vi "tester.vi"() -> ()   [LabVIEW 2020]
uses:
  <vilib>/Utility/miscctls.llb/LVSelectionTypeDef.ctl
panel:
  out "Missmatches 3":T1[](array[typedef])
  out "Common":string="asssd"
  out "Missmatches 2":T1[](array[typedef])
  in  "Reference":string="asd"
  in  "Target":string="asssd"
  in  "String":string
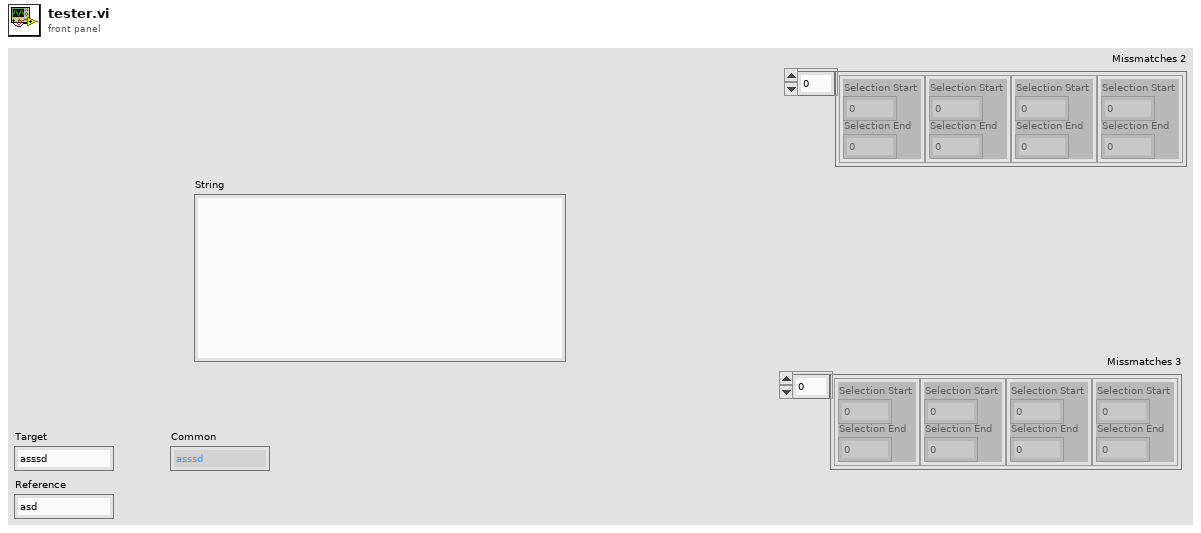
[diagram p1: front panel]
types:
  T1 = typedef "LVSelectionTypeDef.ctl" = cluster{"Selection Start":u32, "Selection End":u32}
  T2 = cluster{"Text.Selection":T1, "Text.Text Colors:Text Color":u32}[]
  T3 = cluster{"Selection Start":u32, "Selection End":u32}[]
  T4 = cluster{"Text.Selection":cluster{"Selection Start":u32, "Selection End":u32}, "Text.Text Colors:Text Color":u32}
  T5 = cluster{"Selection Start":u32, "Selection End":u32}
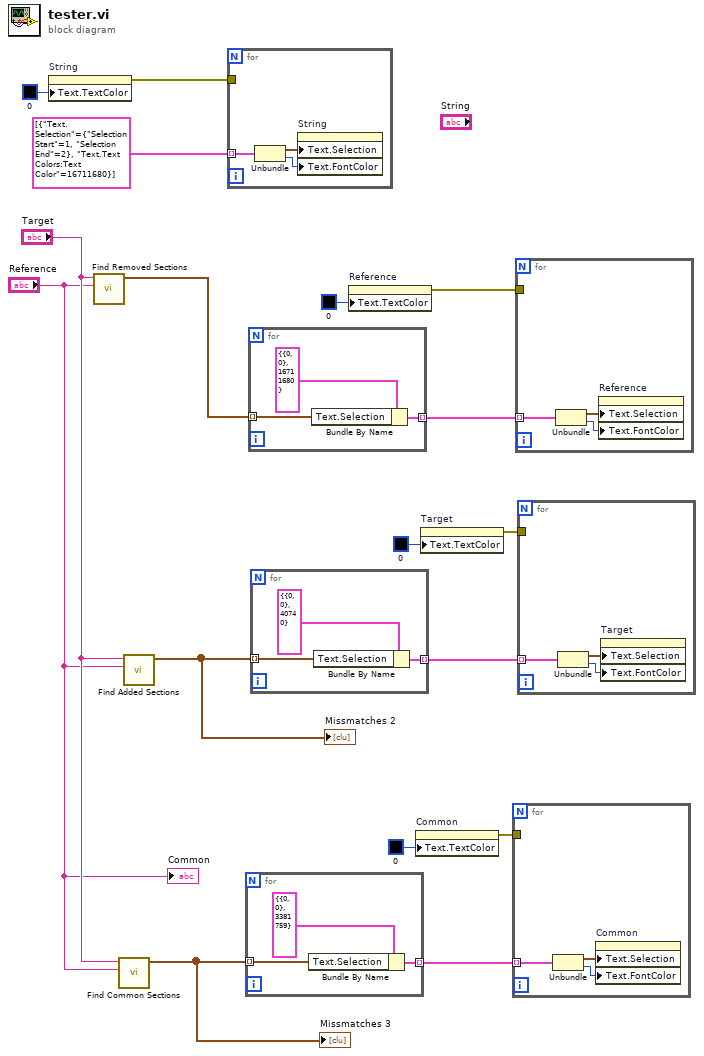
[diagram p0: block diagram]
diagram:
  n1 = property on="String" class="Str"("Text.TextColor"=u32 0 ("Text.Text Colors:Text Color")) -> (error out=w15:errorcluster)  [unwired: 2 in, 1 out]
  n2 = call "Find Removed Sections.vi"("Reference"="Reference", "Target"="Target") -> ("Sections in Reference"=w7:T3)  [unwired: 9 in]
  n3 = call "Find Common Sections.vi"("Reference"="Reference", "Target"="Target") -> ("Sections in Reference"=w6:T3)  [unwired: 9 in]
  "Missmatches 3" <- w6
  n4 = call "Find Added Sections.vi"("Reference"="Reference", "Target"="Target") -> ("Sections in Target"=w11:T3)  [unwired: 9 in]
  "Missmatches 2" <- w11
  n5 = for {
    tunnel: T2 [{"Text.Selection"={"Selection Start"=1, "Selection End"=2}, "Text.Text Colors:Text Color"=16711680}] ("Colors") -> [w20] mode=indexing
    tunnel: w15 -> [_]
    n6 = Unbundle(w20) -> ("Text.Selection"=w19:T1, "Text.Text Colors:Text Color"=w18:u32)
    n7 = property on="String" class="Str"("Text.Selection"=w19, "Text.FontColor"=w18) -> ()  [unwired: 2 in, 2 out]
  }
  n8 = for {
    tunnel: w6 -> [w22] mode=indexing
    tunnel: [w21] -> w5 mode=indexing
    n9 = Bundle By Name(cluster=T4 {"Text.Selection"={"Selection Start"=0, "Selection End"=0}, "Text.Text Colors:Text Color"=3381759} ("Colors"), "Text.Selection"=w22) -> (w21:T4)
  }
  n10 = for {
    tunnel: w7 -> [w25] mode=indexing
    tunnel: [w24] -> w10 mode=indexing
    n11 = Bundle By Name(cluster=T4 {"Text.Selection"={"Selection Start"=0, "Selection End"=0}, "Text.Text Colors:Text Color"=16711680} ("Colors"), "Text.Selection"=w25) -> (w24:T4)
  }
  n12 = for {
    tunnel: w11 -> [w28] mode=indexing
    tunnel: [w27] -> w12 mode=indexing
    n13 = Bundle By Name(cluster=T4 {"Text.Selection"={"Selection Start"=0, "Selection End"=0}, "Text.Text Colors:Text Color"=40740} ("Colors"), "Text.Selection"=w28) -> (w27:T4)
  }
  n14 = property on="Reference" class="Str"("Text.TextColor"=u32 0 ("Text.Text Colors:Text Color")) -> (error out=w8:errorcluster)  [unwired: 2 in, 1 out]
  n15 = property on="Common" class="Str"("Text.TextColor"=u32 0 ("Text.Text Colors:Text Color")) -> (error out=w3:errorcluster)  [unwired: 2 in, 1 out]
  n16 = property on="Target" class="Str"("Text.TextColor"=u32 0 ("Text.Text Colors:Text Color")) -> (error out=w14:errorcluster)  [unwired: 2 in, 1 out]
  n17 = for {
    tunnel: w5 -> [w30] mode=indexing
    tunnel: w3 -> [_]
    n18 = Unbundle(w30) -> ("Text.Selection"=w32:T5, "Text.Text Colors:Text Color"=w31:u32)
    n19 = property on="Common" class="Str"("Text.Selection"=w32, "Text.FontColor"=w31) -> ()  [unwired: 2 in, 2 out]
  }
  n20 = for {
    tunnel: w10 -> [w33] mode=indexing
    tunnel: w8 -> [_]
    n21 = Unbundle(w33) -> ("Text.Selection"=w35:T5, "Text.Text Colors:Text Color"=w34:u32)
    n22 = property on="Reference" class="Str"("Text.Selection"=w35, "Text.FontColor"=w34) -> ()  [unwired: 2 in, 2 out]
  }
  n23 = for {
    tunnel: w12 -> [w36] mode=indexing
    tunnel: w14 -> [_]
    n24 = Unbundle(w36) -> ("Text.Selection"=w38:T5, "Text.Text Colors:Text Color"=w37:u32)
    n25 = property on="Target" class="Str"("Text.Selection"=w38, "Text.FontColor"=w37) -> ()  [unwired: 2 in, 2 out]
  }
  "Common" <- "Reference"
